vi "FindPath.vi"(8 "Wall Left?":bool=TRUE, 9 "dt":dbl, 10 "Lidar Angles":dbl[](array[numeric])=[-119.6484375, -119.296875, -118.9453125, -118.59375, -118.2421875, -117.890625, -117.5390625, -117.1875, -116.8359375, -116.484375, -116.1328125, -115.78125, -115.4296875, -115.078125, -114.7265625, -114.375, -114.0234375, -113.671875, -113.3203125, -112.96875, -112.6171875, -112.265625, -111.9140625, -111.5625, -111.2109375, -110.859375, -110.5078125, -110.15625, -109.8046875, -109.453125, -109.1015625, -108.75, -108.3984375, -108.046875, -107.6953125, -107.34375, -106.9921875, -106.640625, -106.2890625, -105.9375, -105.5859375, -105.234375, -104.8828125, -104.53125, -104.1796875, -103.828125, -103.4765625, -103.125, -102.7734375, -102.421875, -102.0703125, -101.71875, -101.3671875, -101.015625, -100.6640625, -100.3125, -99.9609375, -99.609375, -99.2578125, -98.90625, -98.5546875, -98.203125, -97.8515625, -97.5, -97.1484375, -96.796875, -96.4453125, -96.09375, -95.7421875, -95.390625, -95.0390625, -94.6875, -94.3359375, -93.984375, -93.6328125, -93.28125, -92.9296875, -92.578125, -92.2265625, -91.875, -91.5234375, -91.171875, -90.8203125, -90.46875, -90.1171875, -89.765625, -89.4140625, -89.0625, -88.7109375, -88.359375, -88.0078125, -87.65625, -87.3046875, -86.953125, -86.6015625, -86.25, -85.8984375, -85.546875, -85.1953125, -84.84375, -84.4921875, -84.140625, -83.7890625, -83.4375, -83.0859375, -82.734375, -82.3828125, -82.03125, -81.6796875, -81.328125, -80.9765625, -80.625, -80.2734375, -79.921875, -79.5703125, -79.21875, -78.8671875, -78.515625, -78.1640625, -77.8125, -77.4609375, -77.109375, -76.7578125, -76.40625, -76.0546875, -75.703125, -75.3515625, -75.0, -74.6484375, -74.296875, -73.9453125, -73.59375, -73.2421875, -72.890625, -72.5390625, -72.1875, -71.8359375, -71.484375, -71.1328125, -70.78125, -70.4296875, -70.078125, -69.7265625, -69.375, -69.0234375, -68.671875, -68.3203125, -67.96875, -67.6171875, -67.265625, -66.9140625, -66.5625, -66.2109375, -65.859375, -65.5078125, -65.15625, -64.8046875, -64.453125, -64.1015625, -63.75, -63.3984375, -63.046875, -62.6953125, -62.34375, -61.9921875, -61.640625, -61.2890625, -60.9375, -60.5859375, -60.234375, -59.8828125, -59.53125, -59.1796875, -58.828125, -58.4765625, -58.125, -57.7734375, -57.421875, -57.0703125, -56.71875, -56.3671875, -56.015625, -55.6640625, -55.3125, -54.9609375, -54.609375, -54.2578125, -53.90625, -53.5546875, -53.203125, -52.8515625, -52.5, -52.1484375, -51.796875, -51.4453125, -51.09375, -50.7421875, -50.390625, -50.0390625, -49.6875, -49.3359375, -48.984375, -48.6328125, -48.28125, -47.9296875, -47.578125, -47.2265625, -46.875, -46.5234375, -46.171875, -45.8203125, -45.46875, -45.1171875, -44.765625, -44.4140625, -44.0625, -43.7109375, -43.359375, -43.0078125, -42.65625, -42.3046875, -41.953125, -41.6015625, -41.25, -40.8984375, -40.546875, -40.1953125, -39.84375, -39.4921875, -39.140625, -38.7890625, -38.4375, -38.0859375, -37.734375, -37.3828125, -37.03125, -36.6796875, -36.328125, -35.9765625, -35.625, -35.2734375, -34.921875, -34.5703125, -34.21875, -33.8671875, -33.515625, -33.1640625, -32.8125, -32.4609375, -32.109375, -31.7578125, -31.40625, -31.0546875, -30.703125, -30.3515625, -30.0, -29.6484375, -29.296875, -28.9453125, -28.59375, -28.2421875, -27.890625, -27.5390625, -27.1875, -26.8359375, -26.484375, -26.1328125, -25.78125, -25.4296875, -25.078125, -24.7265625, -24.375, -24.0234375, -23.671875, -23.3203125, -22.96875, -22.6171875, -22.265625, -21.9140625, -21.5625, -21.2109375, -20.859375, -20.5078125, -20.15625, -19.8046875, -19.453125, -19.1015625, -18.75, -18.3984375, -18.046875, -17.6953125, -17.34375, -16.9921875, -16.640625, -16.2890625, -15.9375, -15.5859375, -15.234375, -14.8828125, -14.53125, -14.1796875, -13.828125, -13.4765625, -13.125, -12.7734375, -12.421875, -12.0703125, -11.71875, -11.3671875, -7.5, -7.1484375, -6.796875, -6.4453125, -6.09375, -5.7421875, -5.390625, -5.0390625, -4.6875, -4.3359375, -3.984375, -3.6328125, -3.28125, -2.9296875, -2.578125, -2.2265625, 61.7578125, 62.109375, 62.4609375, 62.8125, 63.1640625, 63.515625, 82.5, 82.8515625, 83.203125, 83.5546875, 83.90625, 84.2578125, 84.609375, 84.9609375, 85.3125, 85.6640625, 86.015625, 86.3671875, 86.71875, 87.0703125, 87.421875, 87.7734375, 88.125, 88.4765625, 88.828125, 89.1796875, 89.53125, 89.8828125, 90.234375, 90.5859375, 90.9375, 91.2890625, 91.640625, 91.9921875, 92.34375, 92.6953125, 93.046875, 93.3984375, 93.75, 94.1015625, 94.453125, 94.8046875, 95.15625, 95.5078125, 95.859375, 96.2109375, 96.5625, 96.9140625, 97.265625, 97.6171875, 97.96875, 98.3203125, 98.671875, 99.0234375, 99.375, 99.7265625, 100.078125, 100.4296875, 100.78125, 101.1328125, 101.484375, 101.8359375, 102.1875, 102.5390625, 102.890625, 103.2421875, 103.59375, 103.9453125, 104.296875, 104.6484375, 105.0, 105.3515625, 105.703125, 106.0546875, 106.40625, 106.7578125, 107.109375, 107.4609375, 107.8125, 108.1640625, 108.515625, 108.8671875, 109.21875, 109.5703125, 109.921875, 110.2734375, 110.625, 110.9765625, 111.328125, 111.6796875, 112.03125, 112.3828125, 112.734375, 113.0859375, 113.4375, 113.7890625, 114.140625, 114.4921875, 114.84375, 115.1953125, 115.546875, 115.8984375, 116.25, 116.6015625, 116.953125, 117.3046875, 117.65625, 118.0078125, 118.359375, 118.7109375, 119.0625, 119.4140625, 119.765625], 11 "Lidar Distances":dbl[](array[numeric])=[57.0, 57.0, 57.0, 66.0, 66.0, 66.0, 66.0, 66.0, 62.0, 61.0, 60.0, 60.0, 60.0, 74.0, 93.0, 736.0, 748.0, 748.0, 736.0, 718.0, 691.0, 656.0, 655.0, 631.0, 602.0, 575.0, 549.0, 507.0, 507.0, 488.0, 481.0, 468.0, 468.0, 457.0, 456.0, 440.0, 437.0, 437.0, 419.0, 405.0, 383.0, 379.0, 376.0, 376.0, 376.0, 369.0, 368.0, 368.0, 360.0, 344.0, 340.0, 333.0, 333.0, 331.0, 327.0, 324.0, 311.0, 305.0, 298.0, 291.0, 291.0, 291.0, 287.0, 281.0, 277.0, 274.0, 273.0, 271.0, 259.0, 259.0, 255.0, 254.0, 251.0, 247.0, 247.0, 247.0, 239.0, 239.0, 239.0, 238.0, 227.0, 225.0, 225.0, 224.0, 224.0, 219.0, 209.0, 209.0, 209.0, 209.0, 208.0, 208.0, 208.0, 208.0, 208.0, 208.0, 208.0, 200.0, 194.0, 192.0, 191.0, 191.0, 189.0, 189.0, 189.0, 189.0, 189.0, 185.0, 184.0, 180.0, 179.0, 175.0, 179.0, 175.0, 175.0, 174.0, 166.0, 165.0, 164.0, 165.0, 165.0, 160.0, 158.0, 158.0, 157.0, 157.0, 158.0, 158.0, 153.0, 153.0, 146.0, 146.0, 146.0, 151.0, 151.0, 154.0, 151.0, 142.0, 142.0, 142.0, 142.0, 138.0, 138.0, 135.0, 135.0, 135.0, 135.0, 131.0, 131.0, 133.0, 131.0, 133.0, 133.0, 137.0, 135.0, 135.0, 133.0, 133.0, 128.0, 128.0, 128.0, 128.0, 128.0, 123.0, 122.0, 122.0, 122.0, 122.0, 126.0, 127.0, 127.0, 130.0, 127.0, 127.0, 125.0, 127.0, 125.0, 125.0, 125.0, 124.0, 124.0, 125.0, 129.0, 129.0, 129.0, 128.0, 127.0, 125.0, 125.0, 125.0, 125.0, 125.0, 124.0, 124.0, 125.0, 124.0, 124.0, 125.0, 125.0, 125.0, 126.0, 126.0, 126.0, 124.0, 122.0, 122.0, 124.0, 129.0, 129.0, 129.0, 127.0, 126.0, 120.0, 120.0, 120.0, 119.0, 119.0, 119.0, 119.0, 121.0, 121.0, 125.0, 125.0, 125.0, 121.0, 121.0, 121.0, 121.0, 121.0, 124.0, 127.0, 125.0, 125.0, 125.0, 124.0, 124.0, 124.0, 129.0, 129.0, 129.0, 128.0, 128.0, 128.0, 128.0, 128.0, 128.0, 127.0, 124.0, 123.0, 124.0, 124.0, 127.0, 130.0, 130.0, 127.0, 129.0, 125.0, 125.0, 126.0, 127.0, 127.0, 127.0, 129.0, 127.0, 129.0, 124.0, 129.0, 130.0, 130.0, 126.0, 132.0, 131.0, 129.0, 129.0, 131.0, 129.0, 129.0, 135.0, 135.0, 135.0, 136.0, 136.0, 136.0, 136.0, 131.0, 127.0, 127.0, 127.0, 127.0, 129.0, 129.0, 127.0, 125.0, 127.0, 125.0, 122.0, 122.0, 121.0, 121.0, 121.0, 214.0, 270.0, 340.0, 3556.0, 3639.0, 3690.0, 3709.0, 3777.0, 3777.0, 178.0, 78.0, 78.0, 78.0, 89.0, 89.0, 89.0, 81.0, 76.0, 71.0, 64.0, 64.0, 64.0, 66.0, 70.0, 72.0, 55.0, 55.0, 59.0, 55.0, 60.0, 60.0, 817.0, 817.0, 817.0, 820.0, 820.0, 820.0, 812.0, 811.0, 791.0, 791.0, 783.0, 781.0, 772.0, 770.0, 764.0, 764.0, 762.0, 751.0, 740.0, 734.0, 734.0, 734.0, 734.0, 727.0, 717.0, 717.0, 717.0, 717.0, 715.0, 714.0, 704.0, 704.0, 702.0, 704.0, 704.0, 706.0, 706.0, 708.0, 706.0, 706.0, 695.0, 695.0, 692.0, 686.0, 685.0, 681.0, 681.0, 677.0, 675.0, 669.0, 666.0, 666.0, 666.0, 659.0, 659.0, 659.0, 656.0, 659.0, 658.0, 656.0, 657.0, 657.0, 654.0, 651.0, 643.0, 640.0, 642.0, 640.0, 640.0, 632.0, 642.0, 632.0, 628.0, 628.0, 624.0, 623.0, 617.0, 617.0, 617.0, 617.0, 612.0, 607.0, 607.0, 600.0, 588.0, 584.0, 580.0, 576.0, 571.0, 568.0, 565.0, 556.0, 551.0, 529.0, 498.0, 268.0, 94.0, 62.0, 60.0, 59.0, 59.0, 59.0, 59.0, 59.0, 66.0, 66.0, 66.0]) -> (3 "New wall following distance":dbl=-0.0)   [LabVIEW 2017]
uses:
  Globals/Pose.vi
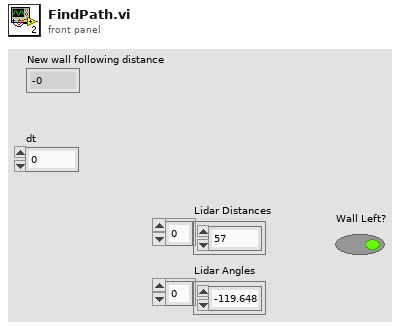
[diagram p1: front panel]
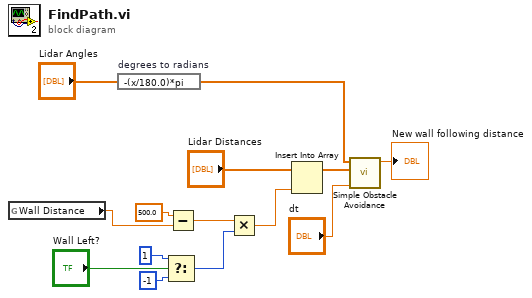
[diagram p0: block diagram]
diagram:
  n1 = global read "Pose.vi" "Wall Distance"() -> (w12:dbl)
  n2 = expression code="-(x/180.0)*pi" "degrees to radians"("Lidar Angles") -> (w2:dbl[])
  n3 = Select(t=1, s="Wall Left?", f=-1) -> (s? t:f=w9:i32)
  n4 = Subtract(x=500.0, y=w12) -> (x-y=w8:dbl)
  n5 = Multiply(x=w8, y=w9) -> (x*y=w3:dbl)
  n6 = Insert Into Array(array="Lidar Distances", new element=w3) -> (w5:dbl[])  [unwired: 1 in]
  n7 = call "Simple Obstacle Avoidance.vi"("dt"="dt", "Lidar Magnitudes"=w5, "Lidar Angles"=w2) -> ("New wall following distance"=→"New wall following distance":dbl)  [unwired: 8 in]
